vi "project_tic_tac_toe.vi"() -> ()   [LabVIEW 2026]
panel:
  in  "Confirm Move":bool
  out "Array 2":string[][](array[string])
  in  "Array":bool[][](array[boolean])
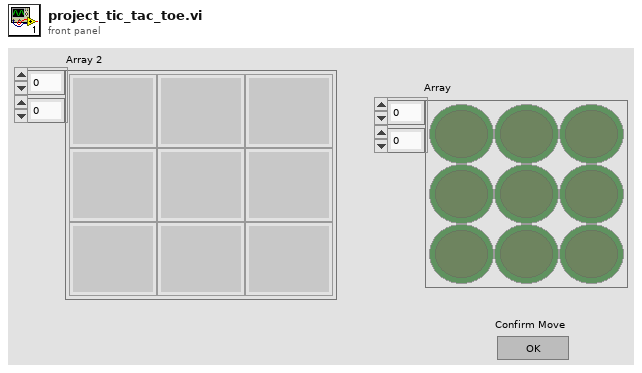
[diagram p1: front panel]
types:
  T1 = enum16{"Exit", "GameOver", "YouWin", "CheckWin", "RobotMove", "PlayerMove", "Init", "CheckWinRobot"}
  T2 = enum16{"Exit", "GameOver", "YouWin", "CheckWin", "RobotMove", "PlayerMove", "Init"}
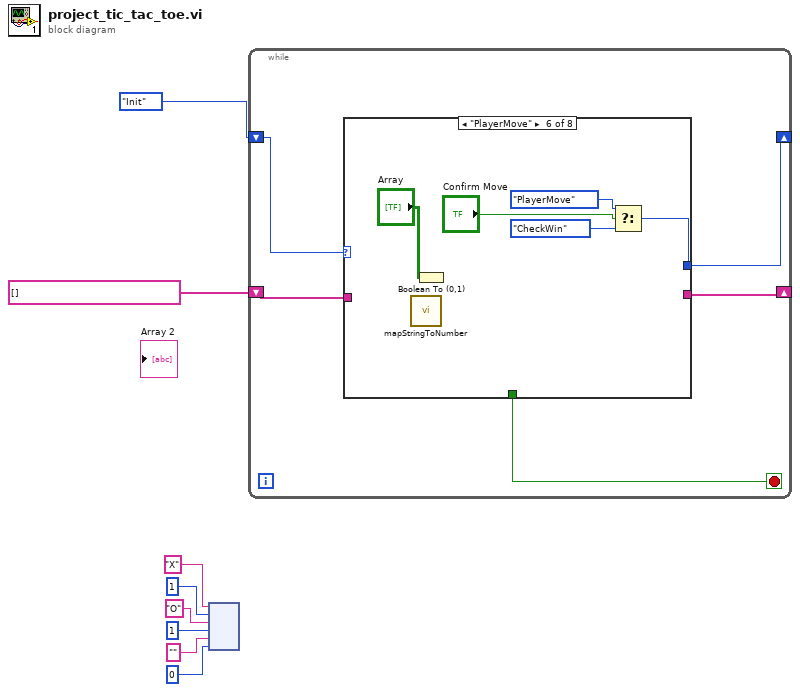
[diagram p0: block diagram]
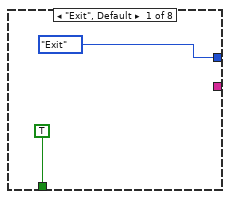
[diagram p2: hidden frame]
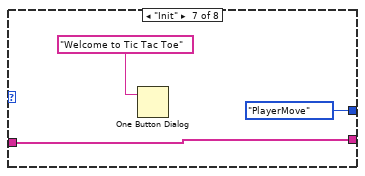
[diagram p7: hidden frame]
diagram:
  n1 = node("X" ("key"), 1 ("value"), "O" ("key"), 1 ("value"), "" ("key"), 0 ("value")) -> ()  [unwired: 1 out]
  n2 = while {
    shift-right: [w12] -> _
    shift-left: T1."Init" -> [w13]
    shift-right: [w10] -> _
    shift-left: string[] [] -> [w9]
    stop <- w11 stop-if-true
    n3 = case shown="\"PlayerMove\"" w13 {
      tunnel: [T2."Exit" _ _ _ _ w18 T2."PlayerMove" _] -> w12
      tunnel: [TRUE _ _ _ _ _ _ _] -> w11
      tunnel: [_ _ _ _ _ _ w22 _] -> w10
      tunnel: w9 -> [_ _ _ _ _ _ w22 _]
      frame "Exit", Default {
      }
      frame "GameOver" {
      }
      frame "YouWin" {
      }
      frame "CheckWin" {
      }
      frame "RobotMove" {
      }
      frame "PlayerMove" {
        n4 = call "mapStringToNumber.vi"() -> ()  [unwired: 11 in, 1 out]
        n5 = Boolean To (0,1)(Boolean="Array") -> (0, 1=w16:i16[][])
        n6 = Select(t=T2."PlayerMove", s="Confirm Move", f=T2."CheckWin") -> (s? t:f=w18:T2)
      }
      frame "Init" {
        n7 = One Button Dialog(message="Welcome to Tic Tac Toe") -> ()  [unwired: 1 in, 1 out]
      }
      frame "CheckWinRobot" {
      }
    }
  }
